vi "PC_PV_profile.vi"() -> ()   [LabVIEW 2016]
panel:
  out "size(s)":i32[](array[numeric])
  out "output array":i32[](array[numeric])
  out "array w/ subset deleted":dbl[][](array[numeric])
  out "array":dbl[][](array[numeric])
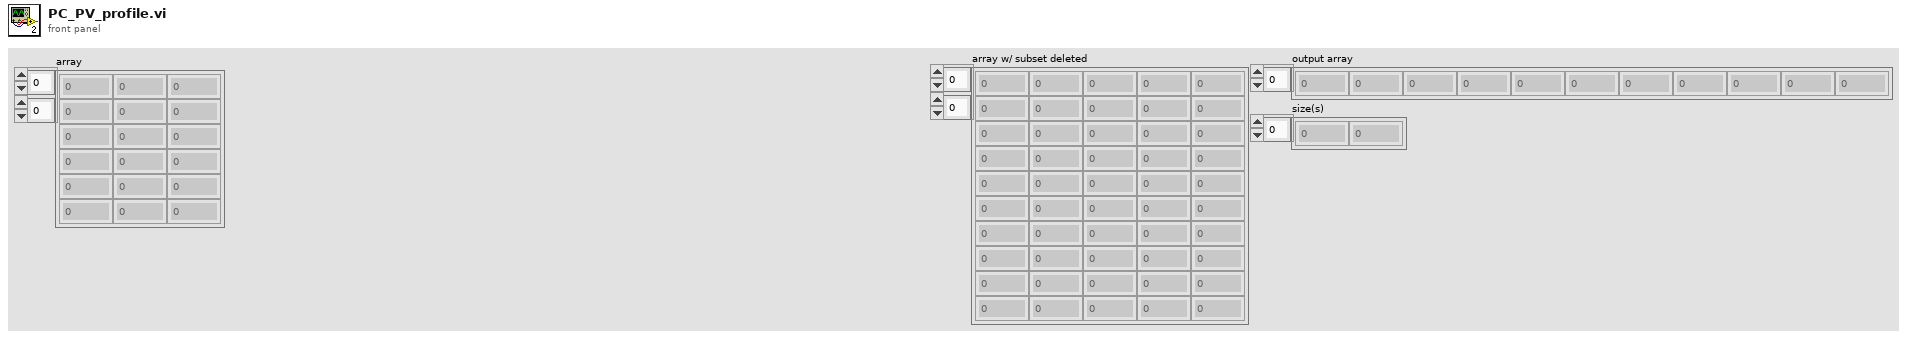
[diagram p1: front panel]
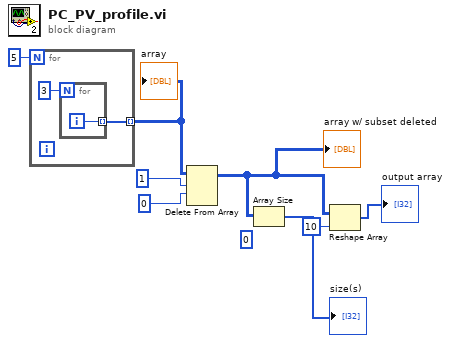
[diagram p0: block diagram]
diagram:
  (unwired) 0 ("dimension size")
  n1 = for {
    N: 5 -> [_]
    tunnel: [w10] -> w6 mode=indexing
    n2 = for {
      N: 3 -> [_]
      tunnel: [w11] -> w10 mode=indexing
      i -> [w11]
    }
  }
  "array" <- w6
  n3 = Delete From Array(array=w6, length=1 ("index"), index (row)=0 ("index")) -> (array with subset deleted=w2:i32[][])  [unwired: 1 in, 1 out]
  "array w/ subset deleted" <- w2
  n4 = Array Size(array=w2) -> (size(s)=→"size(s)":i32[])
  n5 = Reshape Array(w2, 10 ("dimension size")) -> (→"output array":i32[])
